vi "Host - Revert.vi"(8 "error in":errorcluster, 10 "Target IP Address in":string, 11 "Slave Ref in":refnum<k21>) -> (0 "error out":errorcluster, 2 "Target IP Address out":string, 3 "Slave Ref out":refnum<k21>)   [LabVIEW 2011, in "Scan Engine Custom Device.lvlib"]
uses:
  Scan Engine Custom Device.lvlib
  Program Files (x86)/National Instruments/LabVIEW 2011/resource/objmgr/IndComECAT.rc
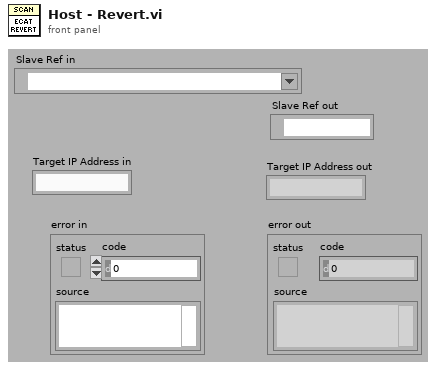
[diagram p1: front panel]
types:
  T1 = enum16{"open", "replace", "create", "open or create", "replace or create", "replace or create with confirmation"}
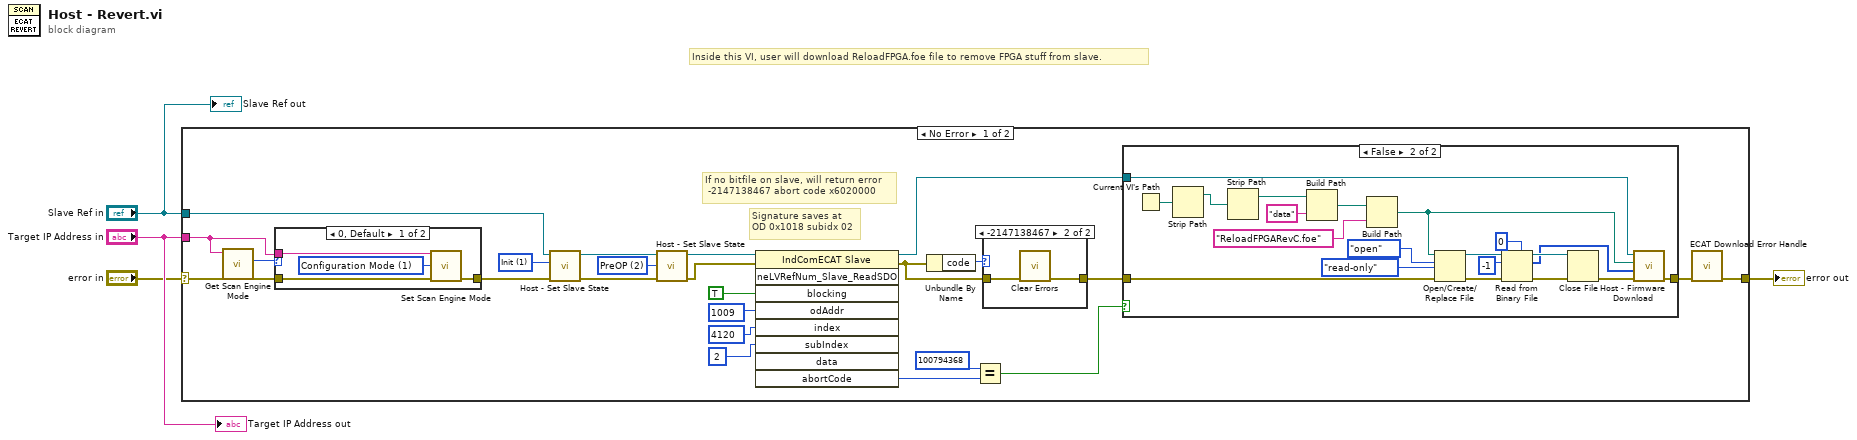
[diagram p0: block diagram]
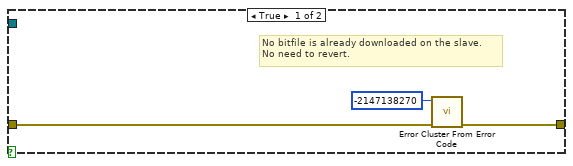
[diagram p3: hidden frame]
diagram:
  # "Inside this VI, user will download ReloadFPGA.foe file to remove FPGA stuff from slave."
  n1 = case shown="No Error" "error in" {
    selector: "error in" -> [w24 w61]
    tunnel: [w28 w61] -> w4
    tunnel: "Target IP Address in" -> [w23 _]
    tunnel: "Slave Ref in" -> [w27 _]
    frame No Error {
      w19 = u32 2 items=["Init"=1, "PreOP"=2, "BootStrap"=3, "SafeOP"=4, "OP"=8] ("slaveState")
      w18 = u32 1 items=["Init"=1, "PreOP"=2, "BootStrap"=3, "SafeOP"=4, "OP"=8] ("slaveState")
      # "If no bitfile on slave, will return error\n -2147138467 abort code x6020000"
      # "Signature saves at \nOD 0x1018 subidx 02"
      n2 = call <vilib>:"Get Scan Engine Mode.vi"("error in (no error)"=w24, "target address (localhost)"=w23) -> ("error out"=w25:errorcluster, "mode"=w26:i32)  [unwired: 8 in]
      n3 = case shown="0, Default" w26 {
        tunnel: w23 -> [w58 _]
        tunnel: w25 -> [w57 w60]
        tunnel: [w56 w60] -> w22
        frame 0, Default {
          w59 = 1 items=["Configuration Mode"=1, "Active Mode"=2] ("mode (Active Mode)")
          n4 = call <vilib>:"Set Scan Engine Mode.vi"("target address (localhost)"=w58, "mode (Active Mode)"=w59, "error in (no error)"=w57) -> ("error out"=w56:errorcluster)  [unwired: 12 in]
        }
        frame 1 {
        }
      }
      n5 = call "Host - Set Slave State.vi"("error in (no error)"=w22, "slaveState"=w18, "Slave Ref in"=w27) -> ("error out"=w21:errorcluster, "Slave Ref out"=w20:refnum<k21>)  [unwired: 5 in, 2 out]
      n6 = call "Host - Set Slave State.vi"("error in (no error)"=w21, "slaveState"=w19, "Slave Ref in"=w20) -> ("error out"=w16:errorcluster, "Slave Ref out"=w17:refnum<k21>)  [unwired: 5 in, 2 out]
      n7 = invoke class="IndComECAT Slave" method="neLVRefNum_Slave_ReadSDO"(reference=w17, error in=w16, "blocking"=TRUE, "odAddr"=u16 1009, "index"=u16 4120, "subIndex"=u8 2) -> (reference out=w13:refnum<k21>, error out=w7:errorcluster, "abortCode"=w6:u32)  [unwired: 3 in, 6 out]
      n8 = Unbundle By Name(w7) -> ("code"=w8:i32)
      n9 = Equal?(x=u32 100794368 ("Numeric 2"), y=w6) -> (x = y?=w15:bool)
      n10 = case shown="-2147138467" w8 {
        tunnel: w7 -> [w30 w32]
        tunnel: [w30 w31] -> w14
        frame 0, Default {
        }
        frame -2147138467 {
          n11 = call <vilib>:"Clear Errors.vi"("error in (no error)"=w32) -> ("error out"=w31:errorcluster)  [unwired: 6 in]
        }
      }
      n12 = case shown="False" w15 {
        tunnel: [w33 w37] -> w29
        tunnel: w14 -> [w34 w55]
        tunnel: w13 -> [_ w36]
        frame True {
          # "No bitfile is already downloaded on the slave.\nNo need to revert."
          n13 = call <vilib>:"Error Cluster From Error Code.vi"("error in (no error)"=w34, "error code (0)"=-2147138270) -> ("error out"=w33:errorcluster)  [unwired: 7 in]
        }
        frame False {
          n14 = Current VI's Path() -> (path=w53:path)
          n15 = Strip Path(path=w53) -> (stripped path=w42:path)  [unwired: 1 out]
          n16 = Strip Path(path=w42) -> (stripped path=w43:path)  [unwired: 1 out]
          n17 = Build Path(base path=w43, name or relative path="data") -> (appended path=w41:path)
          n18 = Build Path(base path=w41, name or relative path="ReloadFPGARevC.foe") -> (appended path=w39:path)
          n19 = Open/Create/Replace File(file path (use dialog)=w39, error in=w55, operation (0:open)=T1."open", access (0:read/write)=enum16{"read/write", "read-only", "write-only"}."read-only") -> (refnum out=w49:refnum<file>, error out=w50:errorcluster)  [unwired: 2 in, 1 out]
          n20 = Read from Binary File(5:u8 0, 8:w50, 10:-1 ("count (1)"), 11:w49) -> (0:w47:errorcluster, 2:w40:u8[], 3:w46:refnum<file>)  [unwired: 2 in, 1 out]
          n21 = Close File(refnum=w46, error in=w47) -> (error out=w38:errorcluster)  [unwired: 1 out]
          n22 = call "Host - Firmware Download.vi"("error in (no error)"=w38, "File Byte Array"=w40, "Firmware filename"=w39, "Slave Ref in"=w36) -> ("error out"=w37:errorcluster)  [unwired: 7 in]
        }
      }
      n23 = call "ECAT Download Error Handle.vi"("error in"=w29) -> ("error out"=w28:errorcluster)  [unwired: 10 in]
    }
    frame Error {
    }
  }
  "error out" <- w4
  "Target IP Address out" <- "Target IP Address in"
  "Slave Ref out" <- "Slave Ref in"
